vi "Configure DIO Direction.vi"(0 "RedPitaya connection in":refnum<k5>, 2 "Pin name":string, 3 "Direction":enum16{"Output", "Input"}(ring), 5 "error in":errorcluster, 12 "timeout ms (2000)":i32=2000) -> (14 "RedPitaya connection out":refnum<k5>, 19 "error out":errorcluster)   [LabVIEW 2010, in "RedPitaya.lvlib"]
doc: "Set direction of digital pins to output or input."
uses:
  RedPitaya.lvlib
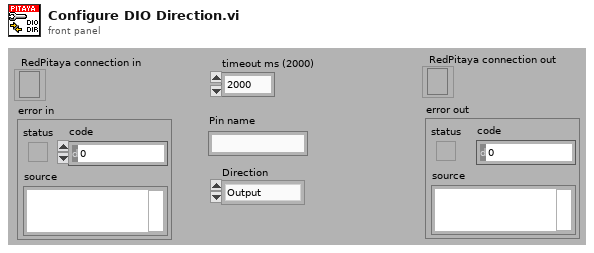
[diagram p1: front panel]
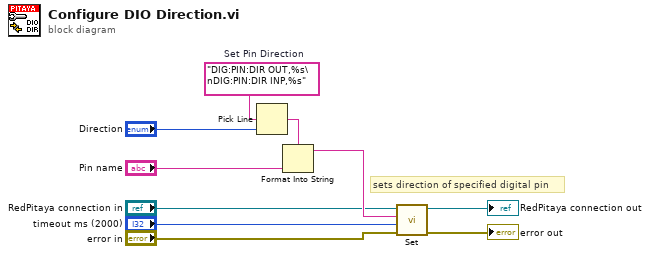
[diagram p0: block diagram]
diagram:
  w4 = "DIG:PIN:DIR OUT,%s\nDIG:PIN:DIR INP,%s"  # Set Pin Direction
  # "sets direction of specified digital pin"
  n1 = Pick Line(multi-line string=w4, line index="Direction") -> (output string=w3:string)  [unwired: 1 in]
  n2 = Format Into String(format string=w3, "Pin name") -> (resulting string=w10:string)  [unwired: 2 in, 1 out]
  n3 = call "Set.vi"("error in"="error in", "timeout ms (2000)"="timeout ms (2000)", "SCPI Message"=w10, "RedPitaya connection in"="RedPitaya connection in") -> ("error out"=→"error out":errorcluster, "RedPitaya connection out"=→"RedPitaya connection out":refnum<k5>)  [unwired: 5 in, 1 out]
